vi "Read Config Data Type from INI file.vi"(4 "Error In":errorcluster) -> (0 "Error Out":errorcluster, 2 "subclass name":string, 3 "subclass relative path":string)   [LabVIEW 2020, in "Config Data.lvlib" / "Config Data.lvclass"]
uses:
  Config Data.lvclass
  typedefs/Data Sources.ctl
  <vilib>/Utility/config.llb/Read Key (String).vi
  <vilib>/Utility/config.llb/Write Key (String).vi
  <vilib>/Utility/config.llb/NI_LVConfig.lvlib
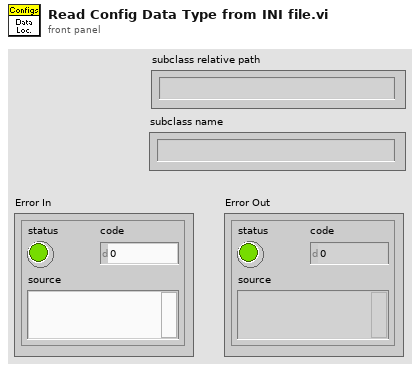
[diagram p1: front panel]
types:
  T1 = typedef "Config Data.lvlib/Config Data.lvclass/Data Sources.ctl" = enum16{"Text", "Jet"}
  T2 = typedef "NI_LVConfig.lvlib/Config Data RefNum.ctl" = refnum<k1>
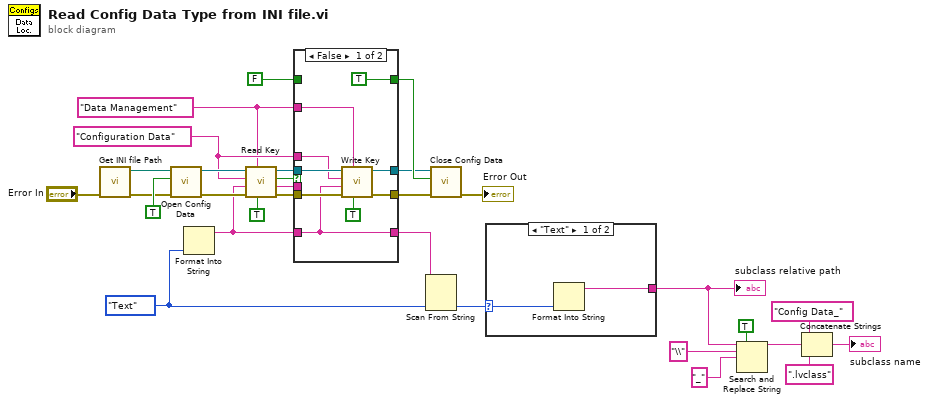
[diagram p0: block diagram]
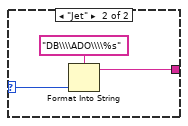
[diagram p2: hidden frame]
diagram:
  w13 = Data_Sources."Text"
  w17 = "Data Management" ("default value")
  w23 = "Configuration Data" ("default value")
  n1 = call "Get INI file Path.vi"("error in (no error)"="Error In") -> ("error out"=w2:errorcluster, "appended path"=w3:path)  [unwired: 5 in]
  n2 = call <vilib>:"Open Config Data.vi"("error in (no error)"=w2, "create file if necessary (T)"=TRUE ("create file if necessary? (T)"), "configuration file path"=w3) -> ("error out"=w28:errorcluster, "refnum"=w27:T2)  [unwired: 6 in, 1 out]
  n3 = Format Into String(w13) -> (resulting string=w15:string)  [unwired: 3 in, 1 out]
  n4 = call-poly <vilib>:"Read Key.vi"("read raw string? (F)"=TRUE, "section"=w17, "error in (no error)"=w28, "default value"=w15, "key"=w23, "refnum"=w27) -> ("error out"=w24:errorcluster, "value"=w22:string, "found?"=w26:bool, "refnum out"=w25:T2)  [unwired: 2 out]
  n5 = case shown="False" w26 {
    tunnel: w25 -> [w38 w42]
    tunnel: w17 -> [w37 _]
    tunnel: w24 -> [w39 w43]
    tunnel: [w34 w43] -> w20
    tunnel: [w35 w42] -> w18
    tunnel: w23 -> [w36 _]
    tunnel: w22 -> [_ w40]
    tunnel: FALSE ("write configuration file? (T)") -> [_ w41]
    tunnel: [TRUE ("write configuration file? (T)") w41] -> w19
    tunnel: w15 -> [w32 _]
    tunnel: [w32 w40] -> w14
    frame False {
      n6 = call-poly <vilib>:"Write Key.vi"("write raw string? (F)"=TRUE ("read raw string? (F)"), "section"=w37, "error in (no error)"=w39, "value"=w32, "key"=w36, "refnum"=w38) -> ("error out"=w34:errorcluster, "refnum out"=w35:T2)  [unwired: 4 out]
    }
    frame True {
    }
  }
  n7 = Scan From String(input string=w14, default 1=w13) -> (output 1=w12:T1)  [unwired: 3 in, 3 out]
  n8 = call <vilib>:"Close Config Data.vi"("error in (no error)"=w20, "write file if changed (T)"=w19, "refnum"=w18) -> ("error out"=→"Error Out":errorcluster)  [unwired: 8 out]
  n9 = case shown="\"Text\"" w12 {
    selector: w12 -> [w45 w48]
    tunnel: [w44 w47] -> w4
    frame "Text" {
      n10 = Format Into String(w45) -> (resulting string=w44:string)  [unwired: 3 in, 1 out]
    }
    frame "Jet" {
      n11 = Format Into String(format string="DB\\\\ADO\\\\%s", w48) -> (resulting string=w47:string)  [unwired: 2 in, 1 out]
    }
  }
  "subclass relative path" <- w4
  n12 = Search and Replace String(replace all?=TRUE ("replace all? (F)"), input string=w4, search string="\\", replace string="_" ("replace string (\"\")")) -> (result string=w5:string)  [unwired: 4 in, 3 out]
  n13 = Concatenate Strings("Config Data_", w5, ".lvclass" ("string")) -> (→"subclass name":string)
